vi "Sensor information.vi"(8 "error in (no error)":errorcluster, 10 "Table":string[][](table)) -> (0 "error in (no error) 2":errorcluster)   [LabVIEW 2015]
uses:
  Control Button/Exit.ctl
  Control Button/Save.ctl
  <vilib>/Utility/miscctls.llb/LVRowAndColumnTypeDef.ctl
panel:
  in  "stop":T1
  in  "Save Button":T2
  out "Active Cell:Active Cell":T3
  # "Sensor Information"
  # "Sensor Name & Unit"
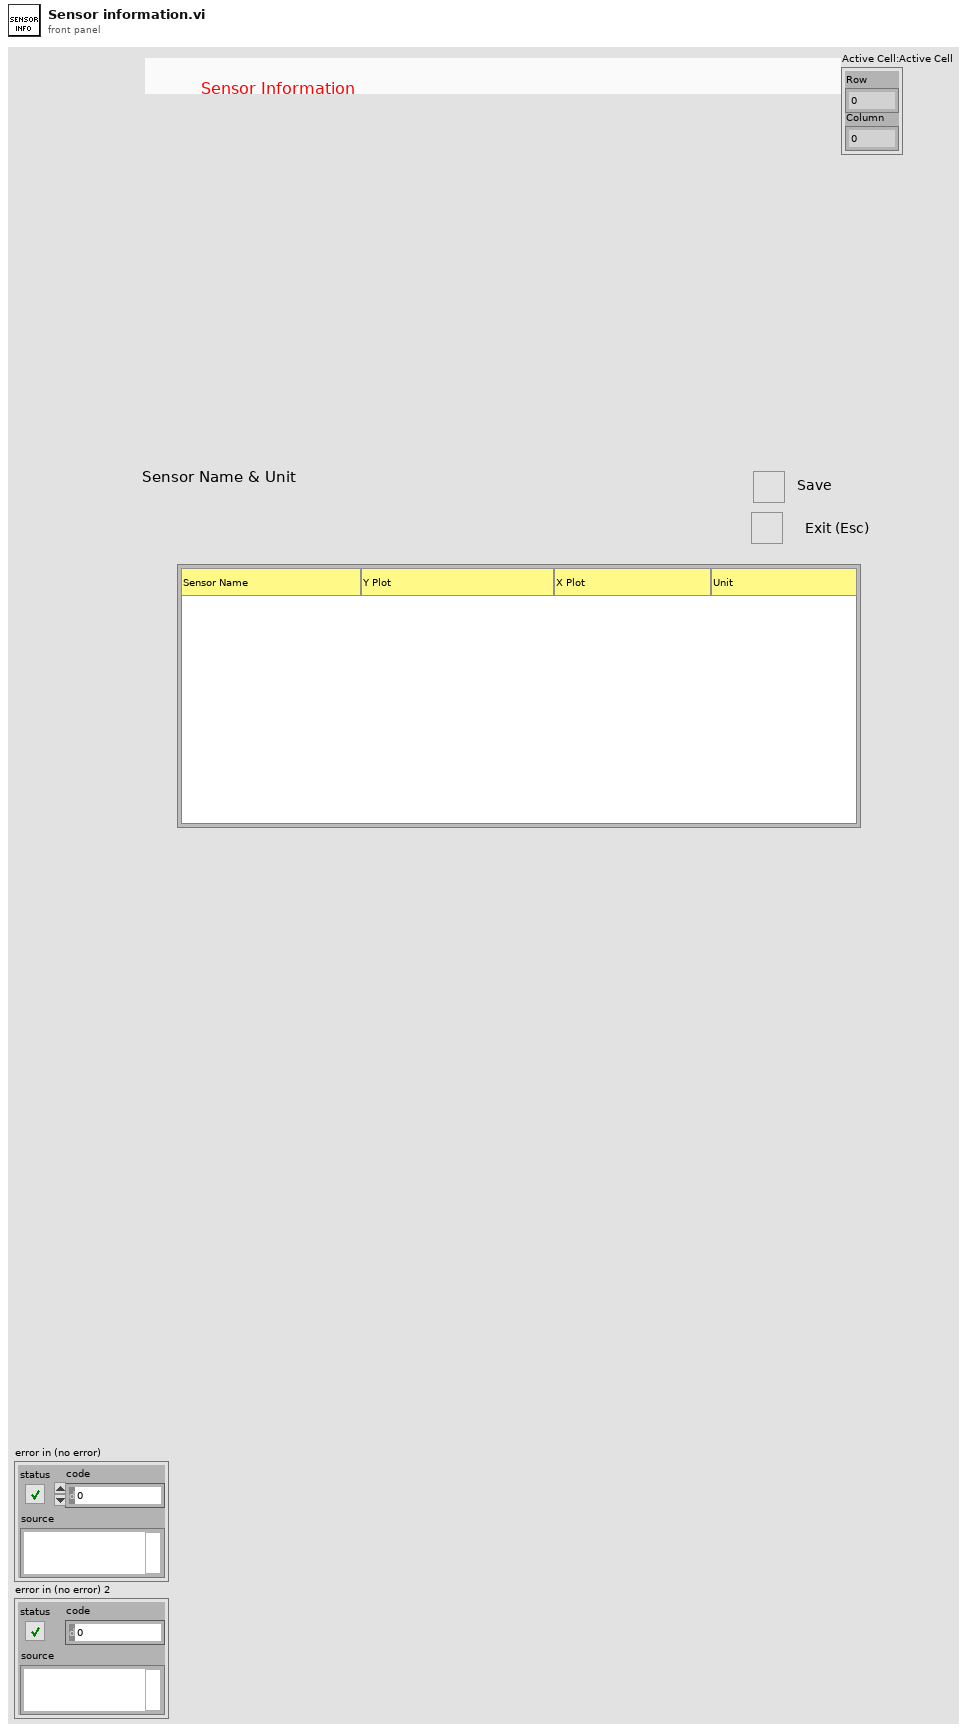
[diagram p1: front panel]
types:
  T1 = typedef "Exit.ctl" = bool
  T2 = typedef "Save.ctl" = bool
  T3 = typedef "LVRowAndColumnTypeDef.ctl" = cluster{"Row":i32, "Column":i32}
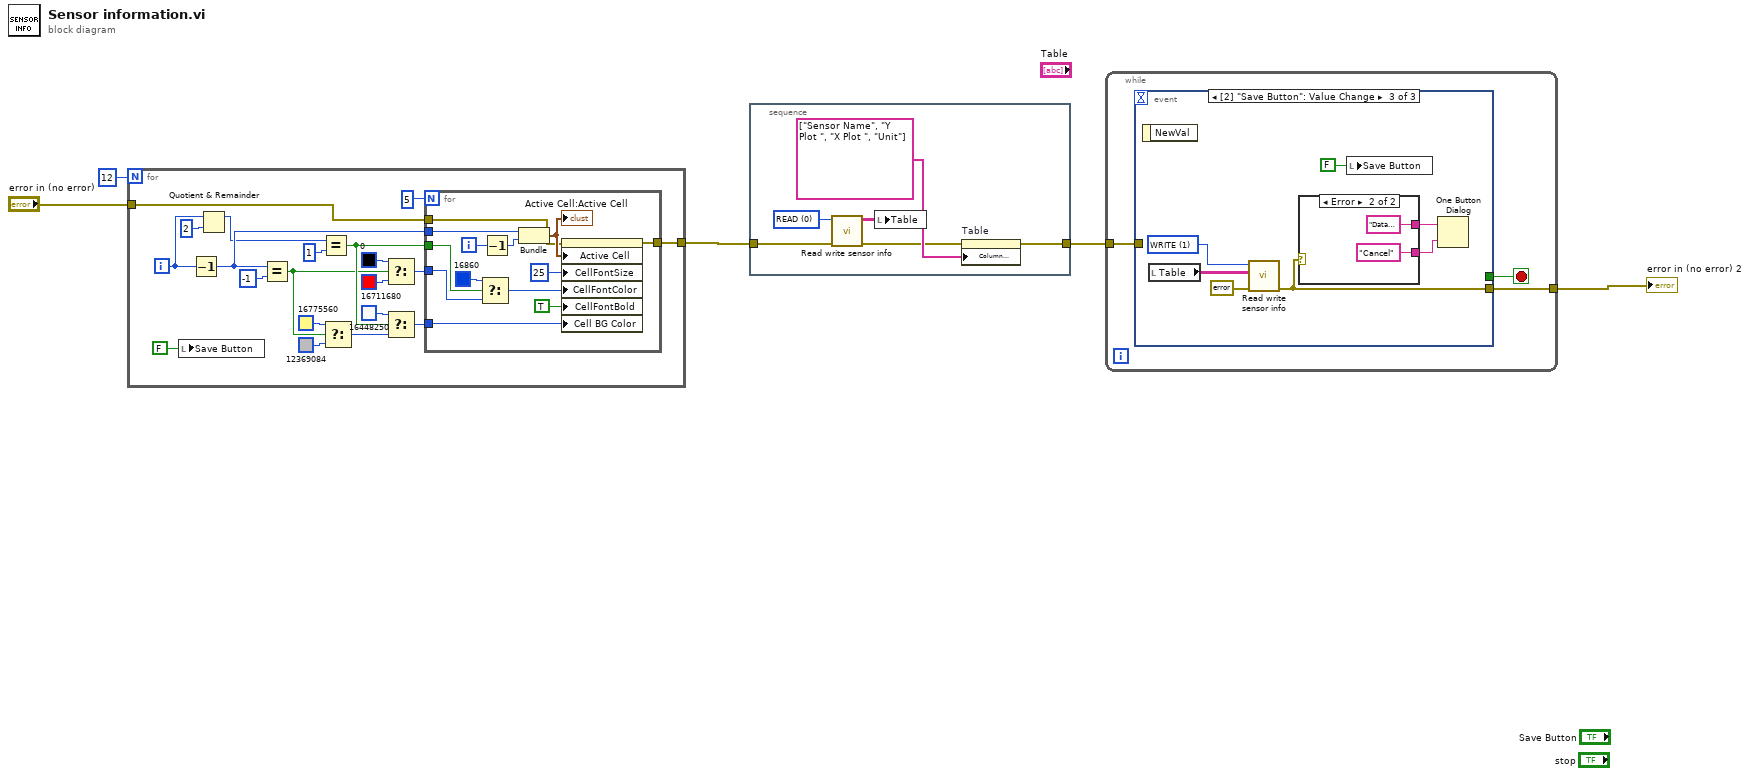
[diagram p0: block diagram]
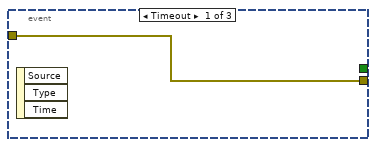
[diagram p2: hidden frame]
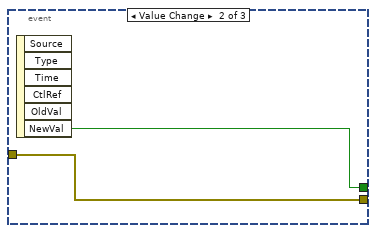
[diagram p3: hidden frame]
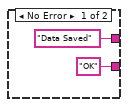
[diagram p4: hidden frame]
diagram:
  n1 = for {
    N: 12 -> [_]
    tunnel: [w8] -> w2
    tunnel: "error in (no error)" -> [w7]
    i -> [w20]
    n2 = local write "Save Button"(FALSE ("Save Button")) -> ()
    n3 = Decrement(x=w20) -> (x-1=w18:i32)
    n4 = Quotient & Remainder(x=w20, y=2) -> (x-y*floor(x/y)=w14:i32)  [unwired: 1 out]
    n5 = Equal?(x=w18, y=-1) -> (x = y?=w11:bool)
    n6 = Equal?(x=w14, y=1) -> (x = y?=w13:bool)
    n7 = Select(t=u32 16775560 ("Color Box"), s=w11, f=u32 12369084 ("Color Box")) -> (s? t:f=w15:u32)
    n8 = Select(t=u32 0 ("Color Box"), s=w11, f=u32 16711680 ("Color Box")) -> (s? t:f=w9:u32)
    n9 = Select(t=u32 16448250 ("Color Box"), s=w13, f=w15) -> (s? t:f=w21:u32)
    n10 = for {
      N: 5 -> [_]
      tunnel: w21 -> [w33]
      tunnel: w18 -> [w37]
      tunnel: w13 -> [w30]
      tunnel: w9 -> [w29]
      tunnel: [w27] -> w8
      tunnel: w7 -> [w26]
      i -> [w36]
      n11 = Select(t=u32 16860 ("Color Box"), s=w30, f=w29) -> (s? t:f=w28:u32)
      n12 = Decrement(x=w36) -> (x-1=w32:i32)
      n13 = Bundle(w37, w32) -> (w35:cluster{i32, i32})  [unwired: 1 in]
      "Active Cell:Active Cell" <- w35
      n14 = property on="Table" class="Tbl (strict)"(error in=w26, "Active Cell"=w35, "CellFontSize"=u32 25 ("Active Cell:Cell Font:Size"), "CellFontColor"=w28, "CellFontBold"=TRUE ("Active Cell:Cell Font:Bold"), "Cell BG Color"=w33) -> (error out=w27:errorcluster)  [unwired: 1 in, 1 out]
    }
  }
  n15 = stacked-sequence {
    tunnel: [w43] -> w5
    tunnel: w2 -> [w40]
    frame #0 {
      w42 = u16 0 items=["READ", "WRITE"] ("Read/Write")
      n16 = call "Read write sensor info.vi"("error in (no error)"=w40, "Read/Write"=w42) -> ("error out"=w39:errorcluster, "Table Control out"=w41:string[][])  [unwired: 8 in]
      n17 = local write "Table"(w41) -> ()
      n18 = property on="Table" class="Tbl (strict)"(error in=w39, "Column Headers[]"=string[] ["Sensor Name", "Y Plot ", "X Plot ", "Unit"] ("Table Control")) -> (error out=w43:errorcluster)  [unwired: 1 in, 1 out]
    }
  }
  n19 = while {
    tunnel: w5 -> [w47]
    tunnel: [w46] -> w4
    stop <- w45 stop-if-true
    n20 = event shown="[2] \"Save Button\": Value Change" {
      selector: _ -> [_ _ _]
      dyn-events: _ -> [_ _ _]
      timeout: _ -> [_ _ _]
      tunnel: w47 -> [w48 w49 _]
      tunnel: [w48 w49 w54] -> w46
      tunnel: [_ w50 _] -> w45
      event Timeout {
        n21 = event-data() -> ()  [unwired: 1 in, 3 out]
      }
      event Value Change {
        n22 = event-data() -> ("NewVal"=w50:T1)  [unwired: 1 in, 5 out]
      }
      event Value Change {
        w57 = u16 1 items=["READ", "WRITE"] ("Read/Write")
        n23 = event-data() -> ()  [unwired: 1 in, 1 out]
        n24 = local read "Table"() -> (w51:string[][])
        n25 = call "Read write sensor info.vi"("error in (no error)"=errorcluster {"status"=FALSE, "code"=0, "source"=""}, "Table Control in"=w51, "Read/Write"=w57) -> ("error out"=w54:errorcluster)  [unwired: 7 in, 1 out]
        n26 = case shown="Error" w54 {
          tunnel: ["Data Saved" ("message") "Data Not Saved,Check The File Path" ("message")] -> w53
          tunnel: ["OK" ("button name (\"OK\")") "Cancel" ("button name (\"OK\")")] -> w52
          frame No Error {
          }
          frame Error {
          }
        }
        n27 = local write "Save Button"(FALSE ("Save Button")) -> ()
        n28 = One Button Dialog(message=w53, button name ("OK")=w52) -> ()  [unwired: 1 out]
      }
    }
  }
  "error in (no error) 2" <- w4
